vi "GetCountdownAction.vi"(9 "PrevStatus":T1(ring), 10 "CurrentStatus":T1(ring), 11 "CurrentMode":T3(ring)=enum."Auto Disabled") -> (1 "Teleop?":bool, 2 "Action":T2)   [LabVIEW 2013]
doc: "Decides what action the timer should take. The possible actions are:\n-Start: when the robot switches from disabled to enabled\n-Reset: when the robot switches from enabled to disabled\n-Continue: when the robot remains in enabled mode\n-Idle: when the robot remains in disabled mode"
uses:
  CountdownAction.ctl
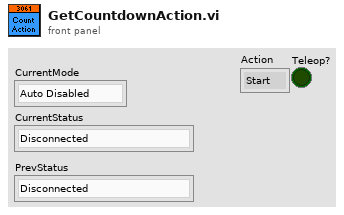
[diagram p1: front panel]
types:
  T1 = enum8{"Disconnected", "E-Stop", "Disabled", "Enabled"}
  T2 = typedef "CountdownAction.ctl" = enum16{"Start", "Reset", "Continue", "Idle"}
  T3 = enum8{"Tele-Op Disabled", "Tele-Op Enabled", "Auto Disabled", "Auto Enabled", "Test Disabled", "Test Enabled", ""}
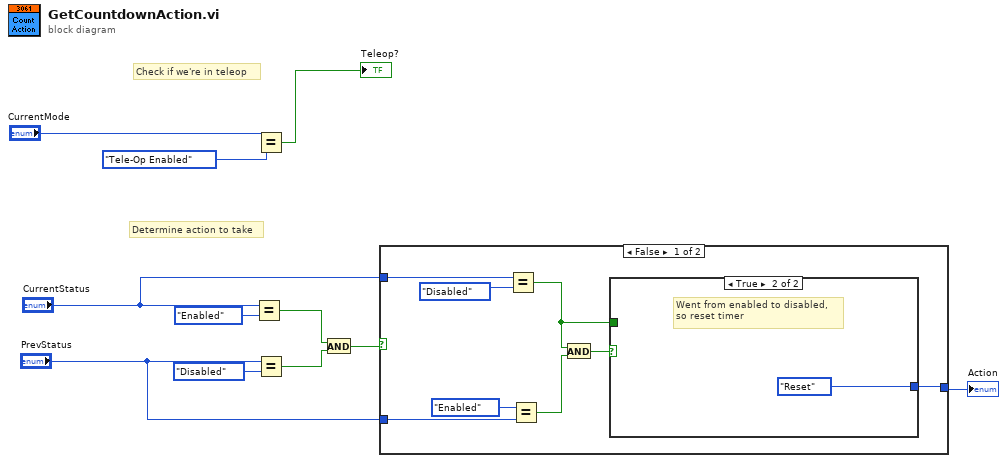
[diagram p0: block diagram]
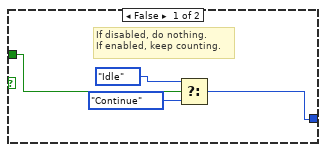
[diagram p2: hidden frame]
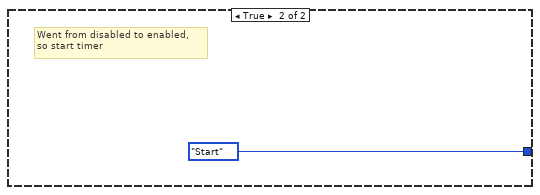
[diagram p3: hidden frame]
diagram:
  # "Determine action to take"
  # "Check if we're in teleop"
  n1 = Equal?(x="CurrentStatus", y=T1."Enabled") -> (x = y?=w6:bool)
  n2 = Equal?(x="CurrentMode", y=T3."Tele-Op Enabled") -> (x = y?=→"Teleop?":bool)
  n3 = Equal?(x="PrevStatus", y=T1."Disabled") -> (x = y?=w5:bool)
  n4 = And(x=w6, y=w5) -> (x .and. y?=w4:bool)
  n5 = case shown="False" w4 {
    tunnel: [w14 CountdownAction."Start" ("Action")] -> w3
    tunnel: "CurrentStatus" -> [w13 _]
    tunnel: "PrevStatus" -> [w19 _]
    frame False {
      n6 = Equal?(x=w13, y=T1."Disabled") -> (x = y?=w12:bool)
      n7 = Equal?(x=T1."Enabled", y=w19) -> (x = y?=w15:bool)
      n8 = And(x=w12, y=w15) -> (x .and. y?=w16:bool)
      n9 = case shown="True" w16 {
        tunnel: [w20 CountdownAction."Reset" ("Action")] -> w14
        tunnel: w12 -> [w23 _]
        frame False {
          # "If disabled, do nothing.\nIf enabled, keep counting."
          n10 = Select(t=CountdownAction."Idle" ("Action"), s=w23, f=CountdownAction."Continue") -> (s? t:f=w20:T2)
        }
        frame True {
          # "Went from enabled to disabled,\nso reset timer"
        }
      }
    }
    frame True {
      # "Went from disabled to enabled, \nso start timer"
    }
  }
  "Action" <- w3
